vi "Configure Sweep Source.vi"(6 "Sweep Source Type (0: Internal)":i32(ring) items=["Internal", "Switcher", "Time", "None"], 7 "Time Source TimeID (0: ttIntersampleDelay)":i32(ring) items=["ttIntersampleDelay", "ttCorrectedTime"], 8 "error in (no error)":errorcluster, 9 "Internal Parameter ID (\"\")":string="\"\"", 10 "Source Axis (1: swpOuter)":i32(ring)=1 items=["swpInner", "swpOuter"], 11 "VISA resource name":refnum<visa-resource-name>) -> (0 "error out":errorcluster, 3 "VISA resource name out":refnum<visa-resource-name>)   [LabVIEW 2014, in "Stanford Research SR1.lvlib"]
doc: "Configures the specified sweep axis as an internal sweep based on the parameter\nspecified by the string ParamID. The string used in ParamID is precisely the same\nstring seen in the \"Source\" window on the Sweep Controller panel when the sweep\nis configured via the user interface."
uses:
  Stanford Research SR1.lvlib
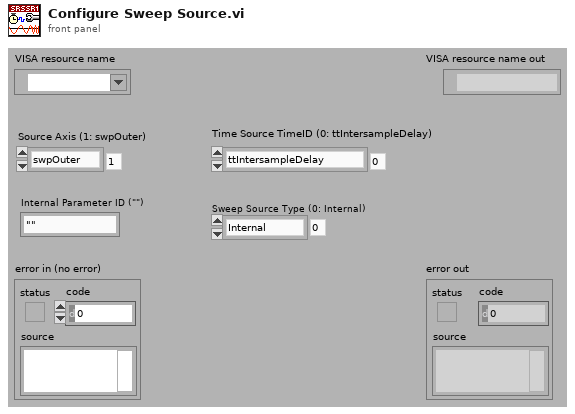
[diagram p1: front panel]
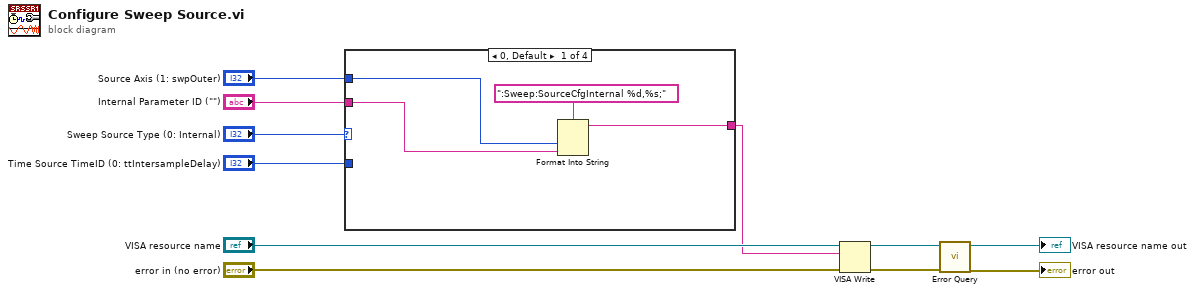
[diagram p0: block diagram]
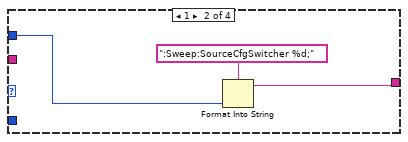
[diagram p2: hidden frame]
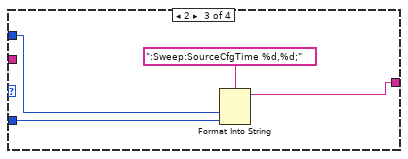
[diagram p3: hidden frame]
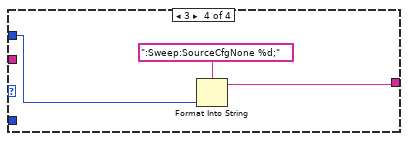
[diagram p4: hidden frame]
diagram:
  n1 = case shown="0, Default" "Sweep Source Type (0: Internal)" {
    tunnel: "Internal Parameter ID (\"\")" -> [w13 _ _ _]
    tunnel: "Time Source TimeID (0: ttIntersampleDelay)" -> [_ _ w20 _]
    tunnel: "Source Axis (1: swpOuter)" -> [w14 w17 w21 w24]
    tunnel: [w12 w16 w19 w23] -> w1
    frame 0, Default {
      n2 = Format Into String(format string=":Sweep:SourceCfgInternal %d,%s;", w14, w13) -> (resulting string=w12:string)  [unwired: 2 in, 1 out]
    }
    frame 1 {
      n3 = Format Into String(format string=":Sweep:SourceCfgSwitcher %d;", w17) -> (resulting string=w16:string)  [unwired: 2 in, 1 out]
    }
    frame 2 {
      n4 = Format Into String(format string=":Sweep:SourceCfgTime %d,%d;", w21, w20) -> (resulting string=w19:string)  [unwired: 2 in, 1 out]
    }
    frame 3 {
      n5 = Format Into String(format string=":Sweep:SourceCfgNone %d;", w24) -> (resulting string=w23:string)  [unwired: 2 in, 1 out]
    }
  }
  n6 = VISA Write(VISA resource name="VISA resource name", write buffer=w1, error in (no error)="error in (no error)") -> (VISA resource name out=w9:refnum<visa-resource-name>, error out=w8:errorcluster)  [unwired: 1 out]
  n7 = call "Error Query.vi"("error in (no error)"=w8, "VISA resource name"=w9) -> ("error out"=→"error out":errorcluster, "VISA resource name out"=→"VISA resource name out":refnum<visa-resource-name>)  [unwired: 6 in, 2 out]
